vi "REPORT_AUDIT_prepare_header_for_csv.vi"(11 "REPORT_AUDIT_all_info":T1) -> (3 "report_header":string[][](array[string]))   [LabVIEW 2020]
uses:
  typedef/REPORT_AUDIT_all_info.ctl
  GEAR/typedef/REPORT_GEAR_statuses.ctl
  _misc/AULocalize/SubVIs/Get Localized Phrase Compact Interface 1D.vi
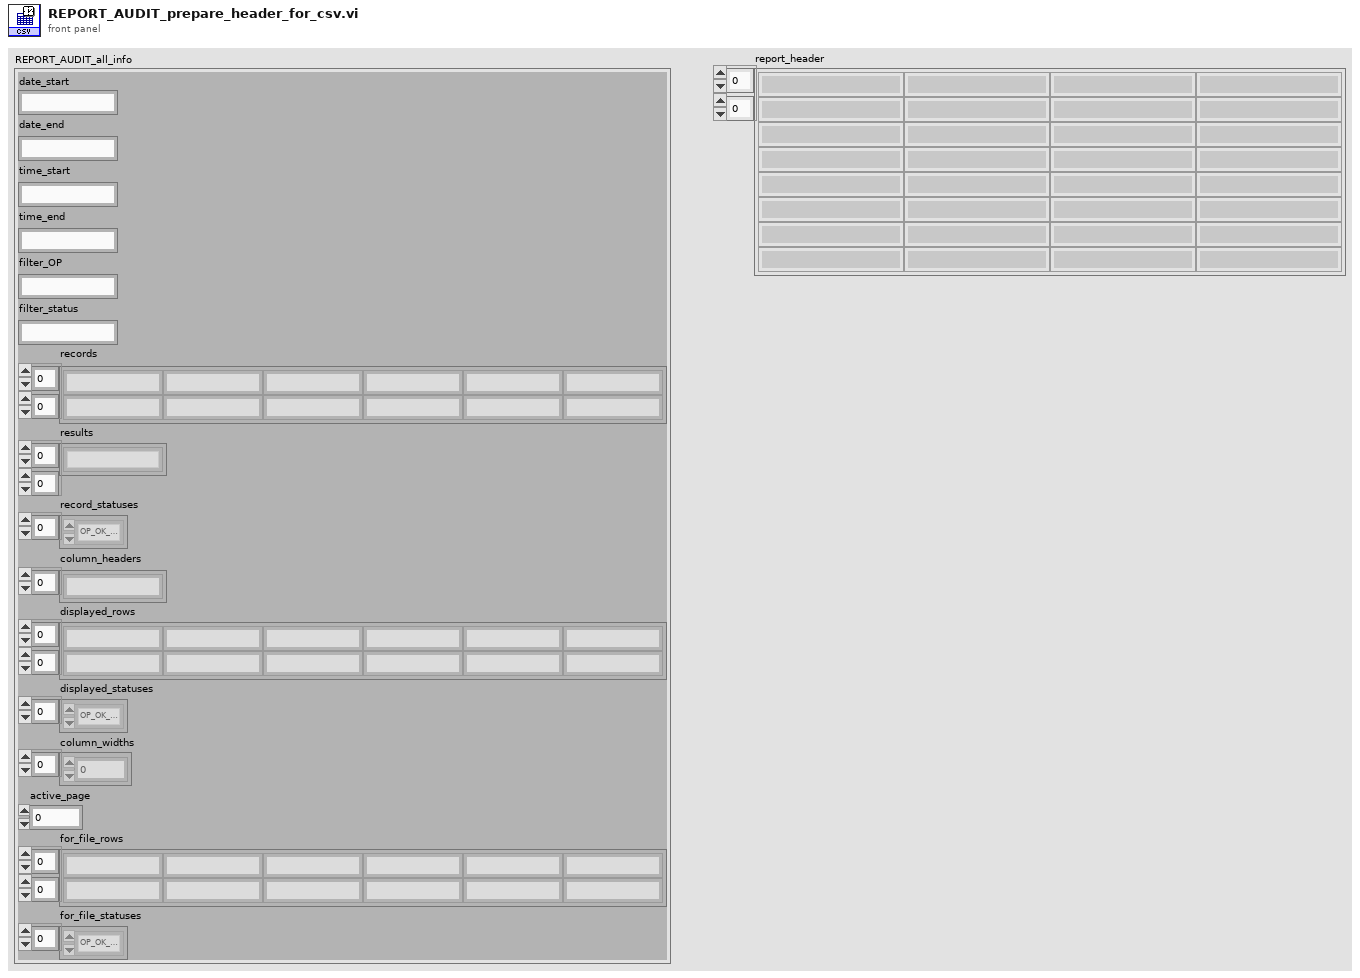
[diagram p1: front panel]
types:
  T1 = typedef "REPORT_AUDIT_all_info.ctl" = cluster{"date_start":string, "date_end":string, "time_start":string, "time_end":string, "filter_OP":string, "filter_status":string, "records":string[][], "results":string[][], "record_statuses":T2[], "column_headers":string[], "displayed_rows":string[][], "displayed_statuses":T2[], "column_widths":i16[], "active_page":i32, "for_file_rows":string[][], "for_file_statuses":T2[]}
  T2 = typedef "REPORT_GEAR_statuses.ctl" = enum16{"OP_OK_hide", "OP_OK_show", "OP_NOK_hide", "OP_NOK_show", "OP_interrupted_hide", "OP_interrupted_show", "OP_in_operation_hide", "OP_in_operation_show", "OP_unexpected_hide", "OP_unexpected_show", "RE_REAL_OK", "RE_REAL_NOK", "RE_STRING", "RE_sub_header", "RE_no_data", "RE_unexpected", "BA_sub_header", "BA_data", "BA_no_data"}
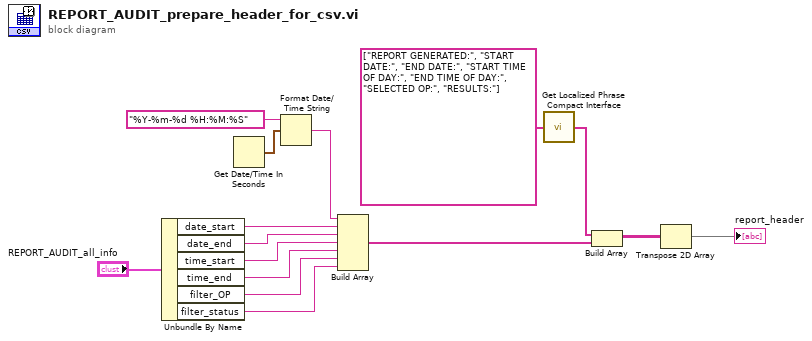
[diagram p0: block diagram]
diagram:
  n1 = Unbundle By Name("REPORT_AUDIT_all_info") -> ("date_start"=w7:string, "date_end"=w6:string, "time_start"=w5:string, "time_end"=w4:string, "filter_OP"=w3:string, "filter_status"=w2:string)
  n2 = Get Date/Time In Seconds() -> (seconds since 1Jan1904=w14:timestamp)
  n3 = Format Date/Time String(time format string (%c)="%Y-%m-%d %H:%M:%S", seconds (now)=w14) -> (date/time string=w8:string)  [unwired: 1 in]
  n4 = Build Array(w8, w7, w6, w5, w4, w3, w2) -> (w9:string[])
  n5 = call-poly "Get Localized Phrase Compact Interface.vi"("Key"=string[] ["REPORT GENERATED:", "START DATE:", "END DATE:", "START TIME OF DAY:", "END TIME OF DAY:", "SELECTED OP:", "RESULTS:"]) -> ("Translated Phrase"=w1:string[])
  n6 = Build Array(w1, w9) -> (w12:string[][])
  n7 = Transpose 2D Array(2D array=w12) -> (transposed array=→"report_header":string[][])
